vi "Module Cleanup.vi"(8 "error in (no error)":errorcluster, 11 "DAQmxAO in":refnum<class "DAQmxAO.lvclass">) -> (0 "error out":errorcluster, 3 "DAQmxAO out":refnum<class "DAQmxAO.lvclass">)   [LabVIEW 2020, in "VolatusDAQ.lvlib" / "DAQmxAO.lvclass"]
uses:
  DAQmxAO.lvclass
  DAQmxAO.lvclass/DAQmxAO.ctl
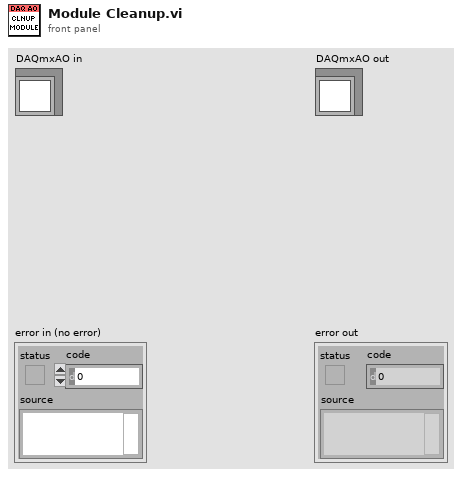
[diagram p1: front panel]
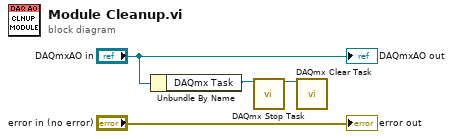
[diagram p0: block diagram]
diagram:
  n1 = Unbundle By Name("DAQmxAO in") -> ("DAQmx Task"=w2:refnum<k21>)
  n2 = call <vilib>:"DAQmx Stop Task.vi"("task/channels in"=w2) -> ("task out"=w1:refnum<k21>)  [unwired: 13 in, 1 out]
  n3 = call <vilib>:"DAQmx Clear Task.vi"("task in"=w1) -> ()  [unwired: 14 in, 1 out]
  "error out" <- "error in (no error)"
  "DAQmxAO out" <- "DAQmxAO in"
